vi "WLAN - RxMeasure - Test.vi"() -> ()   [LabVIEW 2012]
uses:
  TV/RW/Includes/WLAN - TV - OPPO - RW - INC - TV_Rx_Measurements.ctl
  TV/RW/Includes/WLAN - TV - RW - RxPowerLevel.ctl
  <instrlib>/niRFSG/niRFSG.llb/niRFSG Ref Clock Sources.ctl
panel:
  in  "Tab Control":enum32{"Rx_Test Settings", "HW "}(tab)
  in  "Rx Measurements Settings":T1={"Standard"=4, "Channel Bandwidth (Hz)"=40000000.0, "Idle Interval (s)"=0.0001, "MCS Index"=0, "80211n PLCP Frame Format"=0, "Payload Data Length (bytes)"=1024, "OFDM Data Rate (Mbps)"=0, "DSSS Data Rate (Mbps)"=0, "# Packets"=0, "Carrier Frequency(Hz)"=5180000000.0, "Sweep Settings"={"Stop Power Level(dBm)"=-25.0, "Start Power Level(dBm)"=-25.0, "Step Size"=1.0}, "#N_SS"=0} {"DSSS Data Rate (Mbps)" items=["1", "2", "5.5 CCK", "5.5 PBCC", "11 CCK", "11 PBCC", "22", "33"]; "OFDM Data Rate (Mbps)" items=["6", "9", "12", "18", "24", "36", "48", "54"]; "80211n PLCP Frame Format" items=["Mixed Format", "Greenfield Format"]; "Standard" items=["80211A/G/J/P OFDM", "80211B/G DSSS", "80211G DSSSOFDM", "80211N MIMOOFDM", "80211AC MIMOOFDM"]}
  in  "numPackets":i32=5000
  in  "VSG Resource Name":refnum<k15>="rio0"
  in  "Path Loss":dbl
  in  "error in (no error)":errorcluster
  out "error out":errorcluster
  # "GET PACKET COUNT (1)"
  # "PACKET STOP"
  # "PACKET START"
  # "GET PACKET COUNT (2)"
  # "tips: For 11AC, need parameter #N_SS is at least 1"
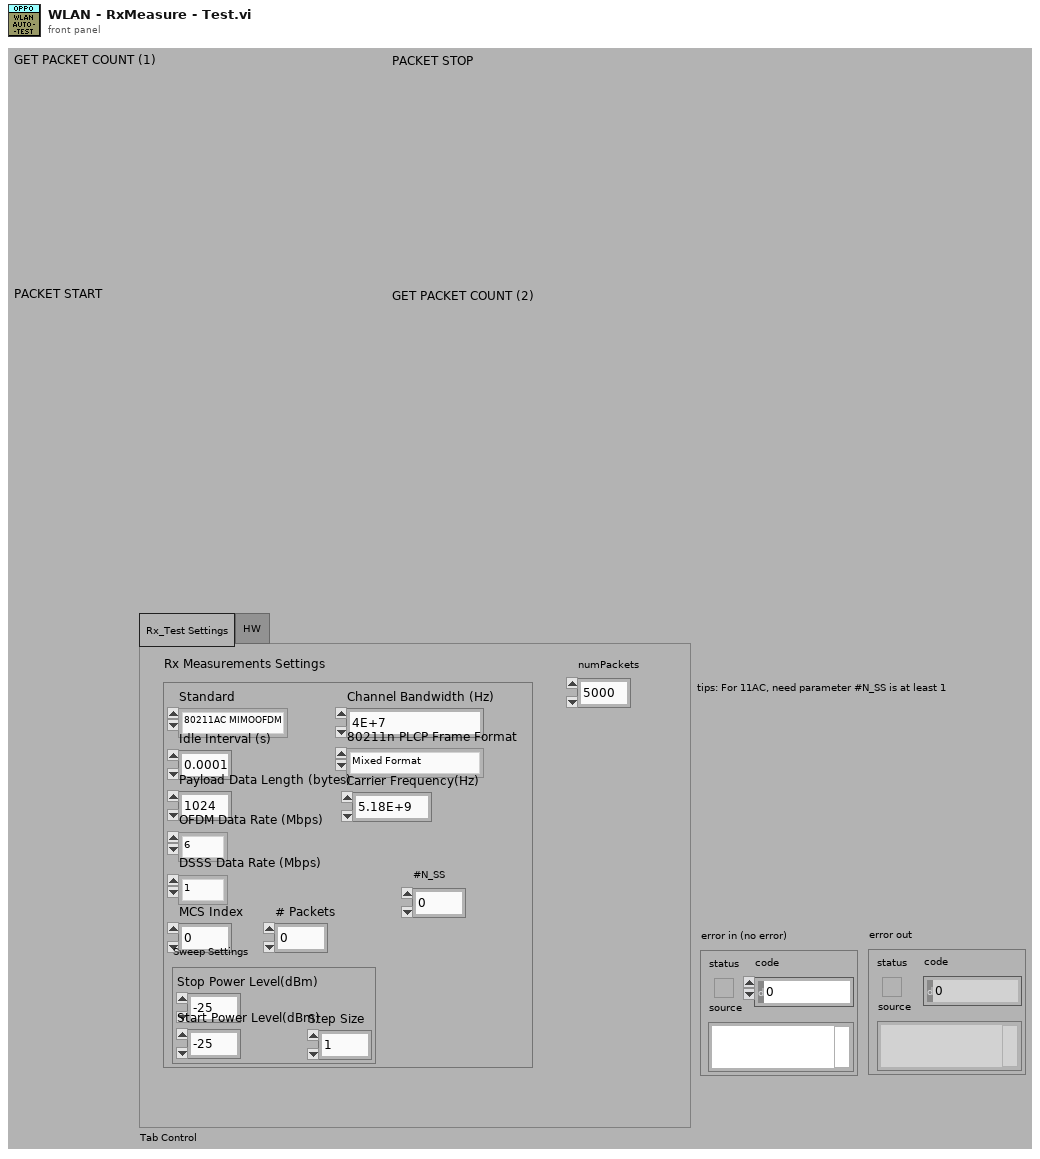
[diagram p1: front panel]
types:
  T1 = typedef "WLAN - TV - OPPO - RW - INC - TV_Rx_Measurements.ctl" = cluster{"Standard":i32, "Channel Bandwidth (Hz)":dbl, "Idle Interval (s)":dbl, "MCS Index":i32, "80211n PLCP Frame Format":i32, "Payload Data Length (bytes)":i32, "OFDM Data Rate (Mbps)":i32, "DSSS Data Rate (Mbps)":i32, "# Packets":i32, "Carrier Frequency(Hz)":dbl, "Sweep Settings":T2, "#N_SS":i32}
  T2 = typedef "WLAN - TV - RW - RxPowerLevel.ctl" = cluster{"Stop Power Level(dBm)":dbl, "Start Power Level(dBm)":dbl, "Step Size":dbl}
  T3 = typedef "niRFSG Ref Clock Sources.ctl" = string
  T4 = typedef "WLAN - TV - RW - INC - Rx_PER_Sweep_Settings.ctl" = cluster{"Wfm_Index":i32, "Power Level Settings":cluster{"Stop Power Level(dBm)":dbl, "Start Power Level(dBm)":dbl, "Step Size":dbl}, "Carrier Frequency(Hz)":dbl}
  T5 = typedef "WLAN - TV - RW - INC - Rx_PER_Wfm_Settings.ctl" = cluster{"Standard":i32, "Channel Bandwidth (Hz)":dbl, "Idle Interval (s)":dbl, "MCS Index":i32, "80211n PLCP Frame Format":i32, "Payload Data Length (bytes)":i32, "OFDM Data Rate (Mbps)":i32, "DSSS Data Rate (Mbps)":i32, "Wfm_Index":i32, "#N_SS":i32}
  T6 = typedef "WLAN - TV - RW - INC - RxTestParameters.ctl" = cluster{"wfm Size in msec":i32, "actual headroom (dB)":dbl, "Size in Samples":i32[], "40M?":bool, "Standard ":i32, "wfm size sec (dbl)":dbl, "dt":dbl, "Channel Bandwidth (Hz)":dbl, "Payload Data Length (bytes)":i32, "80211n PLCP Frame Format":i32, "DSSS Data Rate (Mbps)":i32, "OFDM Data Rate (Mbps)":i32, "MCS Index":i32, "Fc(Hz)":dbl, "#Packets":i32, "#N_SS":i32}
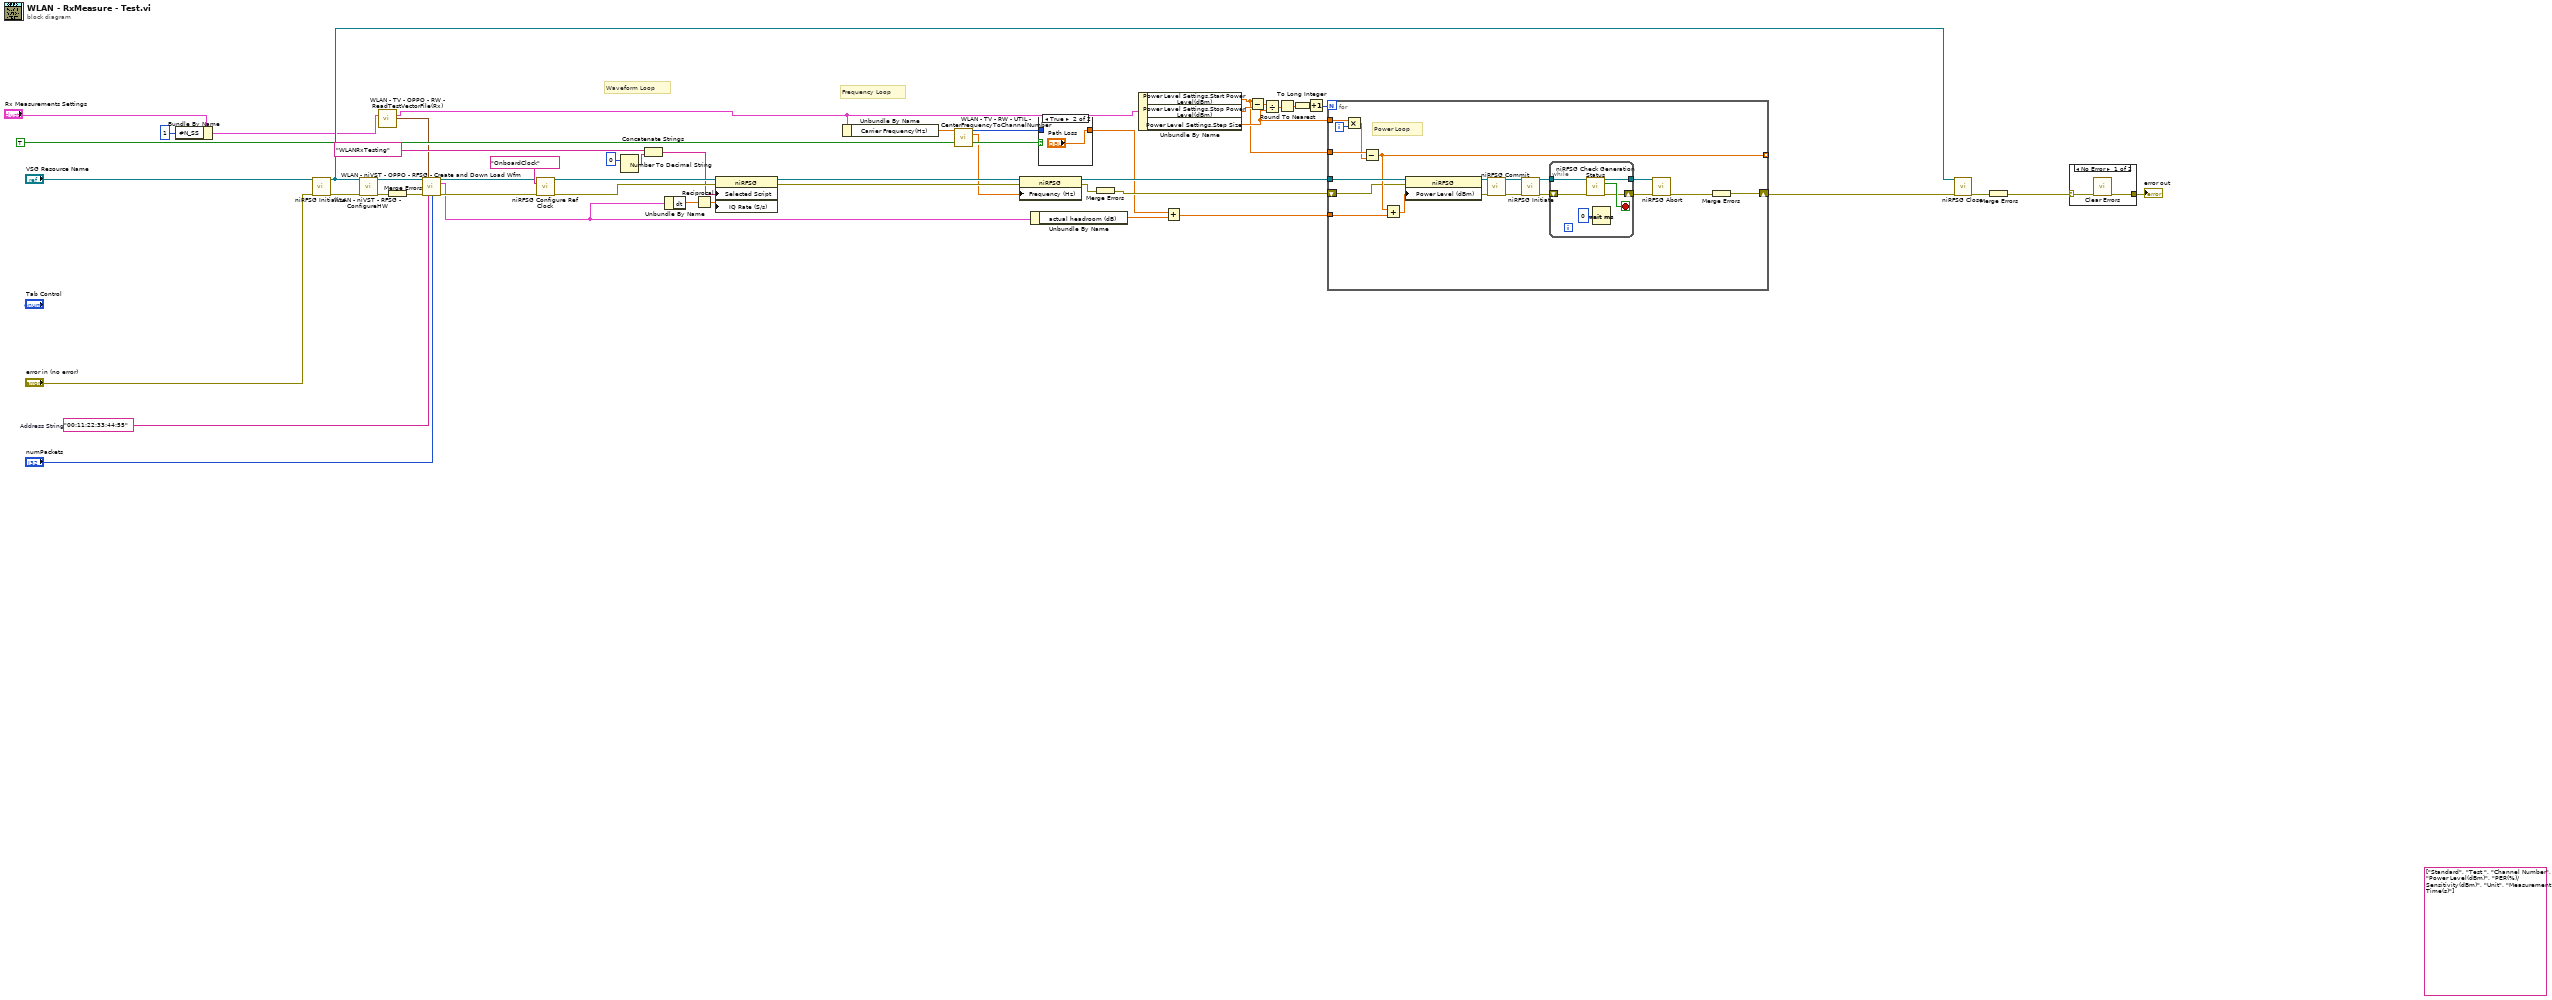
[diagram p0: block diagram]
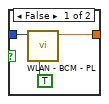
[diagram p2: hidden frame]
diagram:
  w33 = "00:11:22:33:44:55"  # Address String
  (unwired) string[] ["Standard", "Test ", "Channel Number", "Power Level(dBm)", "PER(%)/Sensitivity(dBm)", "Unit", "Measurement Time(s)"]
  # "Frequency Loop"
  # "Waveform Loop"
  n1 = Bundle By Name(cluster="Rx Measurements Settings", "#N_SS"=1) -> (w1:T1)
  n2 = call <instrlib>:"niRFSG Initialize.vi"("resource name"="VSG Resource Name", "error in"="error in (no error)") -> ("instrument handle"=w34:refnum<k15>, "error out"=w46:errorcluster)  [unwired: 12 in]
  n3 = call "WLAN - niVST - RFSG - ConfigureHW.vi"("instrument handle"=w34, "error in"=w46) -> ("instrument handle"=w44:refnum<k15>, "error out"=w38:errorcluster)  [unwired: 12 in]
  n4 = call "WLAN - TV - OPPO - RW - ReadTestVectorFile(Rx).vi"("Rx Measurements Settings"=w1) -> ("PER Sweep Settings"=w5:T4, "Waveform Generation Settings"=w30:T5)  [unwired: 13 in]
  n5 = Merge Errors(w38) -> (w37:errorcluster)
  n6 = call "WLAN - niVST - OPPO - RFSG - Create and Down Load Wfm.vi"("instrument handle"=w44, "Waveform Generation Settings"=w30, "error in"=w37, "Address String"=w33, "numPackets"="numPackets") -> ("instrument handle"=w43:refnum<k15>, "Rx_Test Parameters"=w41:T6, "error out"=w42:errorcluster)  [unwired: 8 in]
  n7 = call <instrlib>:"niRFSG Configure Ref Clock.vi"("instrument handle"=w43, "ref clock source"=T3 "OnboardClock", "error in"=w42) -> ("instrument handle out"=w40:refnum<k15>, "error out"=w39:errorcluster)  [unwired: 11 out]
  n8 = Number To Decimal String(number=0) -> (decimal integer string=w29:string)  [unwired: 1 in]
  n9 = Concatenate Strings("WLANRxTesting" ("Arb:Selected Script"), w29) -> (w28:string)
  n10 = Unbundle By Name(w41) -> ("dt"=w25:dbl)
  n11 = Reciprocal(x=w25) -> (1/x=w26:dbl)
  n12 = property class="niRFSG"(reference=w40, error in=w39, "Selected Script"=w28, "IQ Rate (S/s)"=w26) -> (reference out=w27:refnum<k15>, error out=w24:errorcluster)
  n13 = Unbundle By Name(w5) -> ("Carrier Frequency(Hz)"=w20:dbl)
  n14 = call "WLAN - TV - RW - UTIL - CenterFrequencyToChannelNumber.vi"("Center Frequency(Hz)"=w20) -> ("Coherced Channel Number"=w16:i32, "Coherced Center Frequency (Hz)"=w17:dbl)  [unwired: 13 in]
  n15 = property class="niRFSG"(reference=w27, error in=w24, "Frequency (Hz)"=w17) -> (reference out=w23:refnum<k15>, error out=w22:errorcluster)
  n16 = Unbundle By Name(w41) -> ("actual headroom (dB)"=w18:dbl)
  n17 = case shown="True" TRUE ("PL Manual ?") {
    tunnel: w16 -> [w52 _]
    tunnel: [w51 "Path Loss"] -> w19
    frame False {
      n18 = call "WLAN - BCM - PL.vi"("RX ?"=TRUE, "Channel index"=w52) -> ("PL"=w51:dbl)  [unwired: 9 in]
    }
    frame True {
    }
  }
  n19 = Merge Errors(w22) -> (w21:errorcluster)
  n20 = Unbundle By Name(w5) -> ("Power Level Settings.Start Power Level(dBm)"=w10:dbl, "Power Level Settings.Stop Power Level(dBm)"=w15:dbl, "Power Level Settings.Step Size"=w11:dbl)
  n21 = Add(x=w19, y=w18) -> (x+y=w9:dbl)
  n22 = Subtract(x=w10, y=w15) -> (x-y=w14:dbl)
  n23 = Divide(x=w14, y=w11) -> (x/y=w13:dbl)
  n24 = Round To Nearest(number=w13) -> (nearest integer value=w12:dbl)
  n25 = To Long Integer(number=w12) -> (32bit integer=w7:i32)
  n26 = Increment(x=w7) -> (x+1=w8:i32)
  n27 = for {
    N: w8 -> [_]
    shift-right: [w71] -> w4
    shift-left: w21 -> [w57]
    tunnel: w23 -> [w73]
    tunnel: w11 -> [w63]
    tunnel: w10 -> [w62]
    tunnel: w9 -> [w61]
    tunnel: [w58] -> _ mode=indexing
    i -> [w64]
    # "Power Loop"
    n28 = Multiply(x=w63, y=w64) -> (x*y=w59:dbl)
    n29 = Subtract(x=w62, y=w59) -> (x-y=w58:dbl)
    n30 = Add(x=w58, y=w61) -> (x+y=w60:dbl)
    n31 = property class="niRFSG"(reference=w73, error in=w57, "Power Level (dBm)"=w60) -> (reference out=w68:refnum<k15>, error out=w65:errorcluster)
    n32 = call <instrlib>:"niRFSG Commit.vi"("instrument handle"=w68, "error in"=w65) -> ("instrument handle out"=w67:refnum<k15>, "error out"=w56:errorcluster)  [unwired: 12 in]
    n33 = call <instrlib>:"niRFSG Initiate.vi"("instrument handle"=w67, "error in"=w56) -> ("instrument handle out"=w70:refnum<k15>, "error out"=w66:errorcluster)  [unwired: 12 in]
    n34 = while {
      tunnel: w70 -> [w79]
      tunnel: [w78] -> w69
      shift-right: [w76] -> w55
      shift-left: w66 -> [w75]
      stop <- w77 stop-if-true
      n35 = call <instrlib>:"niRFSG Check Generation Status.vi"("instrument handle"=w79, "error in"=w75) -> ("instrument handle out"=w78:refnum<k15>, "done?"=w77:bool, "error out"=w76:errorcluster)  [unwired: 11 in]
      n36 = Wait (ms)(milliseconds to wait=u32 0) -> ()  [unwired: 1 out]
    }
    n37 = call <instrlib>:"niRFSG Abort.vi"("instrument handle"=w69, "error in"=w55) -> ("error out"=w72:errorcluster)  [unwired: 12 in, 1 out]
    n38 = Merge Errors(w72) -> (w71:errorcluster)
  }
  n39 = call <instrlib>:"niRFSG Close.vi"("instrument handle"=w34, "error in"=w4) -> ("error out"=w49:errorcluster)  [unwired: 13 in]
  n40 = Merge Errors(w49) -> (w31:errorcluster)
  n41 = case shown="No Error" w31 {
    selector: w31 -> [w81 w82]
    tunnel: [w80 w82] -> w47
    frame No Error {
      n42 = call <vilib>:"Clear Errors.vi"("error in (no error)"=w81) -> ("error out"=w80:errorcluster)  [unwired: 6 in]
    }
    frame Error {
    }
  }
  "error out" <- w47
